vi "Reset.vi"(8 "error in (no error)":errorcluster, 10 "reinitialize grating? (F)":bool, 11 "VISA resource name":refnum<visa-resource-name>) -> (0 "error out":errorcluster, 3 "VISA resource name out":refnum<visa-resource-name>)   [LabVIEW 2009, in "JY-SPEX-TRIAX.lvlib"]
doc: "Resets the spectrometer program and optionally re-initializes the grating as well."
uses:
  JY-SPEX-TRIAX.lvlib
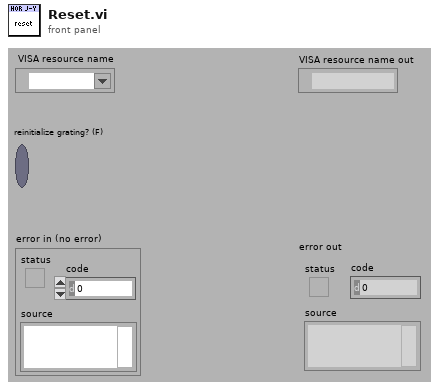
[diagram p1: front panel]
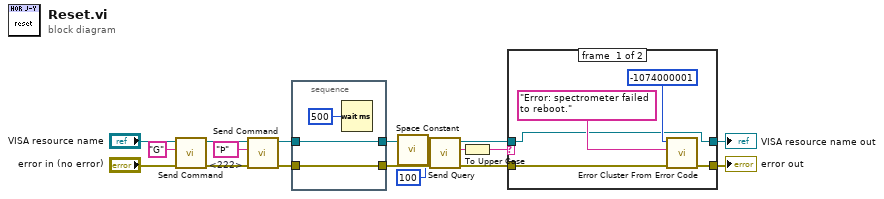
[diagram p0: block diagram]
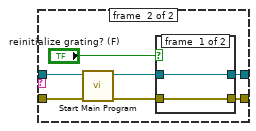
[diagram p2: hidden frame]
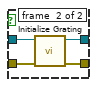
[diagram p3: hidden frame]
diagram:
  w13 = "Þ"  # <222>
  n1 = call "Send Command.vi"("error in (no error)"="error in (no error)", "write buffer"="G", "VISA resource name"="VISA resource name") -> ("error out"=w15:errorcluster, "VISA resource name out"=w17:refnum<visa-resource-name>)  [unwired: 7 out]
  n2 = call "Send Command.vi"("error in (no error)"=w15, "write buffer"=w13, "VISA resource name"=w17) -> ("error out"=w11:errorcluster, "VISA resource name out"=w12:refnum<visa-resource-name>)  [unwired: 7 out]
  n3 = stacked-sequence {
    tunnel: w12 -> [w21]
    tunnel: w11 -> [w20]
    tunnel: [w21] -> w10
    tunnel: [w20] -> w9
    frame #0 {
      n4 = Wait (ms)(milliseconds to wait=u32 500) -> ()  [unwired: 1 out]
    }
  }
  n5 = call <vilib>:"Space Constant.vi"() -> ("String"=w7:string)
  n6 = call "Send Query.vi"("error in (no error)"=w9, "byte count"=u32 100, "write buffer"=w7, "VISA resource name"=w10) -> ("error out"=w3:errorcluster, "read buffer"=w6:string, "VISA resource name out"=w4:refnum<visa-resource-name>)  [unwired: 5 out]
  n7 = To Upper Case(1:w6) -> (0:w5:string)
  n8 = case shown="\"B\", Default" w5 {
    tunnel: w4 -> [w22 w30]
    tunnel: w3 -> [w24 w29]
    tunnel: [w22 w33] -> w2
    tunnel: [w23 w32] -> w1
    frame #0 {
      n9 = call <vilib>:"Error Cluster From Error Code.vi"("error in (no error)"=w24, "error message (\"\")"="Error: spectrometer failed to reboot." ("error message (\"\")"), "error code (0)"=-1074000001) -> ("error out"=w23:errorcluster)  [unwired: 1 in, 5 out]
    }
    frame #1 {
      n10 = call "Start Main Program.vi"("error in (no error)"=w29, "VISA resource name"=w30) -> ("error out"=w27:errorcluster, "VISA resource name out"=w28:refnum<visa-resource-name>)  [unwired: 8 out]
      n11 = case shown="True" "reinitialize grating? (F)" {
        tunnel: w28 -> [w35 w39]
        tunnel: w27 -> [w34 w38]
        tunnel: [w35 w37] -> w33
        tunnel: [w34 w36] -> w32
        frame #0 {
        }
        frame #1 {
          n12 = call "Initialize Grating.vi"("error in (no error)"=w38, "VISA resource name"=w39) -> ("error out"=w36:errorcluster, "VISA resource name out"=w37:refnum<visa-resource-name>)  [unwired: 8 out]
        }
      }
    }
  }
  "error out" <- w1
  "VISA resource name out" <- w2
